vi "Launcher.vi"   [LabVIEW 2020, in "MainWindow.lvlib"]
uses:
  MainWindow.lvlib
  MainWindow/MainWindow.lvclass
  C:/Program Files (x86)/National Instruments/LabVIEW 2020/vi.lib/MGI/Panel Manager/Panel Actor/Panel Actor/Panel Actor.lvclass
  <vilib>/MGI/Panel Manager/Panel/Window Position/Reference Position/Ref Display/Ref Display.lvclass
  C:/Program Files (x86)/National Instruments/LabVIEW 2020/vi.lib/MGI/Panel Manager/Panel/Window Position/Window Position.lvclass
  <vilib>/MGI/Panel Manager/Panel/Window Position/Reference Position/Ref Display/Ref Display.vi
  <vilib>/MGI/Panel Manager/Panel Actor/Panel Actor/Launch Root Panel Window.vi
  <vilib>/MGI/Panel Manager/Panel Actor/Panel Actor/Panel Actor.lvclass
  <vilib>/MGI/Panel Manager/Panel/Panel.lvlib
  C:/Program Files (x86)/National Instruments/LabVIEW 2020/vi.lib/MGI/Panel Manager/Panel/Window Position/Reference Position/Reference Position.lvclass
  C:/Program Files (x86)/National Instruments/LabVIEW 2020/vi.lib/MGI/Panel Manager/Panel/Window Position/Reference Position/Ref Display/Ref Display.lvclass
  C:/Program Files (x86)/National Instruments/LabVIEW 2020/vi.lib/MGI/Monitored Actor/Monitored Actor/Monitored Actor/Monitored Actor.lvclass
  C:/Program Files (x86)/National Instruments/LabVIEW 2020/vi.lib/ActorFramework/Actor/Actor.lvclass
  C:/Users/Test/Git/MGIPanelActors-Exploration/src/MainWindow/MainWindow/MainWindow.lvclass
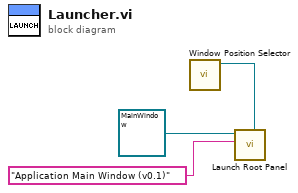
[diagram p0: block diagram]
diagram:
  n1 = call-poly <vilib>:"Window Position Selector.vi"() -> ("Ref Display out"=w1:refnum<class "Ref Display.lvclass">)  [unwired: 10 in, 1 out]
  n2 = call-poly <vilib>:"Launch Root Panel.vi"("Window Position (Maximize First Call)"=w1, "Title"="Application Main Window (v0.1)", "Panel Actor in"=refnum<class "MainWindow.lvclass"> refnum ("MainWindow.lvlib:MainWindow.lvclass")) -> ()  [unwired: 7 in, 2 out]
